vi "Sequence.CheckNameConflicts.vi"(11 "Aliases.All":T1[](array[typedef])) -> (3 "Warning":string)   [LabVIEW 2015, in "Simple Sequence Tools - Editor.lvlib"]
uses:
  Simple Sequence Tools - Editor.lvlib
  Shared/Types/Channel.Properties.ctl
  Shared/Simple Sequence Tools - Shared.lvlib
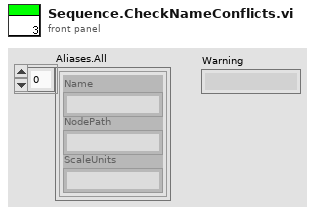
[diagram p1: front panel]
types:
  T1 = typedef "Simple Sequence Tools - Shared.lvlib/Channel.Properties.ctl" = cluster{"Name":string, "NodePath":string, "ScaleUnits":string}
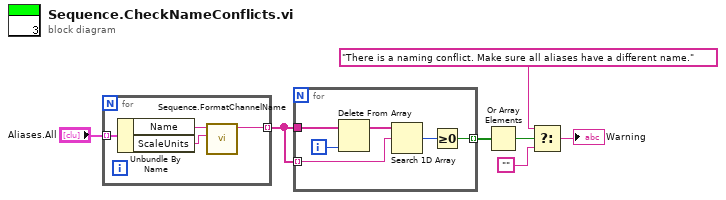
[diagram p0: block diagram]
diagram:
  n1 = for {
    tunnel: "Aliases.All" -> [w9] mode=indexing
    tunnel: [w8] -> w3 mode=indexing
    n2 = Unbundle By Name(w9) -> ("Name"=w10:string, "ScaleUnits"=w11:string)
    n3 = call "Sequence.FormatChannelName.vi"("ScaleUnits"=w11, "Name"=w10) -> ("ChannelName"=w8:string)  [unwired: 9 in]
  }
  n4 = for {
    tunnel: w3 -> [w17]
    tunnel: w3 -> [w14] mode=indexing
    tunnel: [w12] -> w4 mode=indexing
    i -> [w16]
    n5 = Delete From Array(array=w17, index=w16) -> (array with subset deleted=w15:string[])  [unwired: 1 in, 1 out]
    n6 = Search 1D Array(1D array=w15, element=w14) -> (index of element=w13:i32)  [unwired: 1 in]
    n7 = Greater Or Equal To 0?(x=w13) -> (x >= 0?=w12:bool)
  }
  n8 = Or Array Elements(Boolean array=w4) -> (logical OR=w5:bool)
  n9 = Select(t="There is a naming conflict. Make sure all aliases have a different name.", s=w5, f="") -> (s? t:f=→"Warning":string)
